vi "ISMBUS_DecodeModuleTypes.vi"(8 "Fehler (Eingang - kein Fehler)":errorcluster, 11 "ModuleKindIndex":i32) -> (0 "error (Ausgang)":errorcluster caption="error IO", 3 "ModulType String":string)   [LabVIEW 2016]
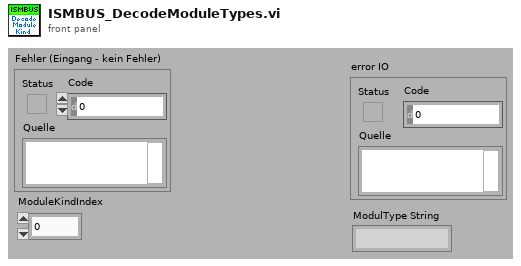
[diagram p1: front panel]
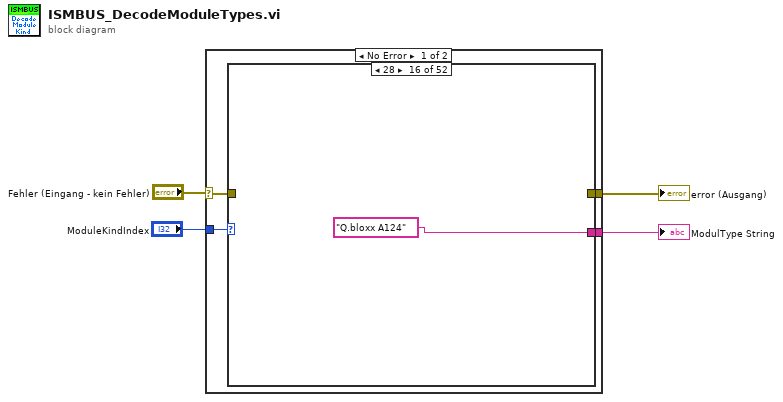
[diagram p0: block diagram]
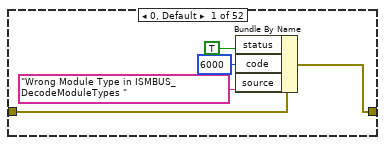
[diagram p2: hidden frame]
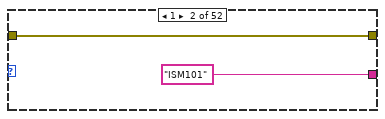
[diagram p3: hidden frame]
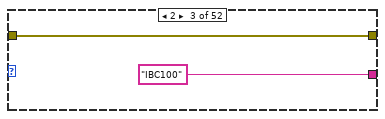
[diagram p4: hidden frame]
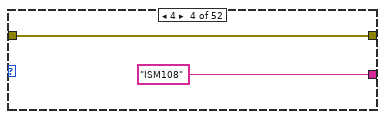
[diagram p5: hidden frame]
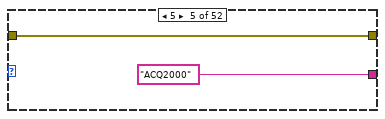
[diagram p6: hidden frame]
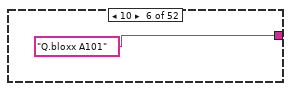
[diagram p7: hidden frame]
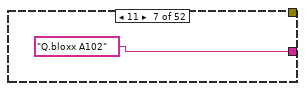
[diagram p8: hidden frame]
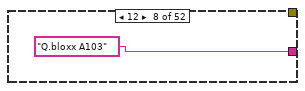
[diagram p9: hidden frame]
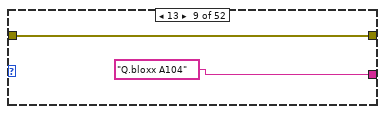
[diagram p10: hidden frame]
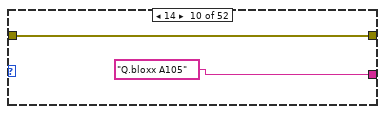
[diagram p11: hidden frame]
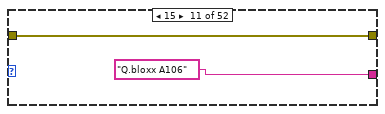
[diagram p12: hidden frame]
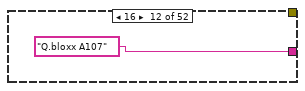
[diagram p13: hidden frame]
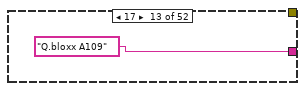
[diagram p14: hidden frame]
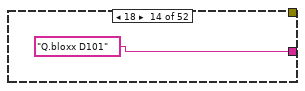
[diagram p15: hidden frame]
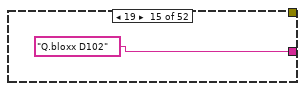
[diagram p16: hidden frame]
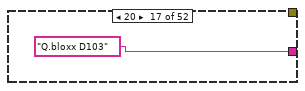
[diagram p17: hidden frame]
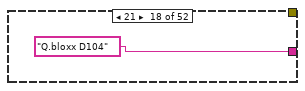
[diagram p18: hidden frame]
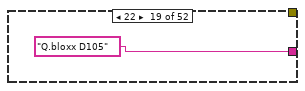
[diagram p19: hidden frame]
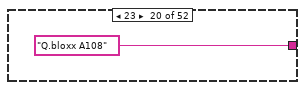
[diagram p20: hidden frame]
diagram:
  n1 = case shown="No Error" "Fehler (Eingang - kein Fehler)" {
    selector: "Fehler (Eingang - kein Fehler)" -> [w6 w104]
    tunnel: "ModuleKindIndex" -> [w8 _]
    tunnel: [w7 _] -> w1
    tunnel: [w5 w104] -> w2
    frame No Error {
      n2 = case shown="28" w8 {
        tunnel: [_ "ISM101" "IBC100" "ISM108" "ACQ2000" "Q.bloxx A101" "Q.bloxx A102" "Q.bloxx A103" "Q.bloxx A104" "Q.bloxx A105" "Q.bloxx A106" "Q.bloxx A107" "Q.bloxx A109" "Q.bloxx D101" "Q.bloxx D102" "Q.bloxx A124" "Q.bloxx D103" "Q.bloxx D104" "Q.bloxx D105" "Q.bloxx A108" "TBLOXX L3" " IDL112" " IDL101" " IDL100" " ISM101" " ISM102" " ISM103" " ITL104" "ISM110" "ISM111" "ISM112" "IDM118" "IDM165" "e.bloxx A1" "e.bloxx A6-1 CF" "e.bloxx A5-1 CR" "e.bloxx A2" "e.bloxx D3 CAN" "e.bloxx A3" "e.bloxx D4" "e.bloxx A4" "e.bloxx A4-1 TC" "e.bloxx A5" "e.bloxx A6-2 CF" "e.bloxx A9" "e.bloxx D3 COM" "e.bloxx D3 SSI" "e.bloxx D1" "e.bloxx D2" "e.bloxx A6-2 DC" "e.reader EX8" "ADL-MXE"] -> w7
        tunnel: w6 -> [w12 w14 w16 w18 w20 _ _ _ w25 w27 w29 _ _ _ _ _ _ _ _ _ w40 w42 w44 w46 w48 w50 w52 w54 w56 w58 w60 w62 w64 w66 w68 w70 w72 w74 w76 w78 w80 w82 w84 w86 w88 w90 w92 w94 w96 w98 w100 w102]
        tunnel: [w13 w14 w16 w18 w20 _ _ _ w25 w27 w29 _ _ _ _ _ _ _ _ _ w40 w42 w44 w46 w48 w50 w52 w54 w56 w58 w60 w62 w64 w66 w68 w70 w72 w74 w76 w78 w80 w82 w84 w86 w88 w90 w92 w94 w96 w98 w100 w102] -> w5
        frame 0, Default {
          n3 = Bundle By Name(cluster=w12, "status"=TRUE, "code"=6000, "source"="Wrong Module Type in ISMBUS_DecodeModuleTypes ") -> (w13:errorcluster)
        }
        frame 1 {
        }
        frame 2 {
        }
        frame 4 {
        }
        frame 5 {
        }
        frame 10 {
        }
        frame 11 {
        }
        frame 12 {
        }
        frame 13 {
        }
        frame 14 {
        }
        frame 15 {
        }
        frame 16 {
        }
        frame 17 {
        }
        frame 18 {
        }
        frame 19 {
        }
        frame 28 {
        }
        frame 20 {
        }
        frame 21 {
        }
        frame 22 {
        }
        frame 23 {
        }
        frame 97 {
        }
        frame 98 {
        }
        frame 99 {
        }
        frame 100 {
        }
        frame 101 {
        }
        frame 102 {
        }
        frame 103 {
        }
        frame 104 {
        }
        frame 110 {
        }
        frame 111 {
        }
        frame 112 {
        }
        frame 118 {
        }
        frame 165 {
        }
        frame 200 {
        }
        frame 201 {
        }
        frame 202 {
        }
        frame 203 {
        }
        frame 204 {
        }
        frame 205 {
        }
        frame 206 {
        }
        frame 207 {
        }
        frame 208 {
        }
        frame 209 {
        }
        frame 210 {
        }
        frame 211 {
        }
        frame 212 {
        }
        frame 213 {
        }
        frame 214 {
        }
        frame 216 {
        }
        frame 217 {
        }
        frame 230 {
        }
        frame 231 {
        }
      }
    }
    frame Error {
    }
  }
  "error (Ausgang)" <- w2
  "ModulType String" <- w1
